vi "Measure Current.vi"(8 "error in":errorcluster, 11 "6700 in":refnum<class "6700.lvclass">) -> (0 "error out":errorcluster, 2 "Current":dbl, 3 "6700 out":refnum<class "6700.lvclass">)   [LabVIEW 2018, in "6700.lvlib" / "6700.lvclass"]
uses:
  6700.lvclass
  6700.lvclass/6700.ctl
  <instrlib>/Agilent N6700 Series/Agilent N6700 Series.lvlib
  builds/Power_Supply.lvlibp/Power Supply.lvclass
  C:/Users/Ron.Dexter.LUMINARTECH/Desktop/builds/Power_Supply.lvlibp/Power Supply.lvclass
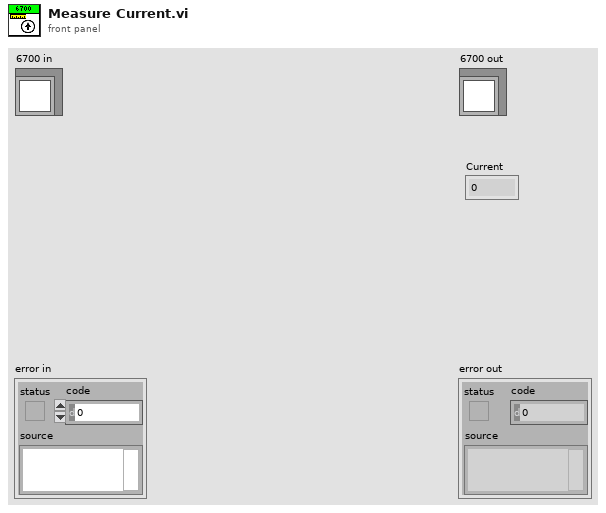
[diagram p1: front panel]
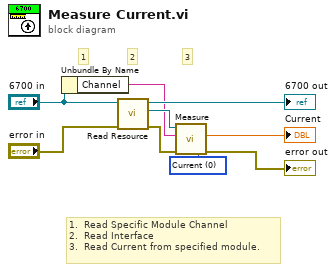
[diagram p0: block diagram]
diagram:
  w4 = 0 items=["Current", "Voltage", "Power"] ("Measurement Type (1: Voltage)")
  # "1.  Read Specific Module Channel \n2.  Read Interface\n3.  Read Current from specified module."
  # "3"
  # "2"
  # "1"
  n1 = Unbundle By Name("6700 in") -> ("Channel"=w1:string)
  n2 = call "Read Resource.vi"("error in"="error in", "Power Supply in"="6700 in") -> ("error out"=w5:errorcluster, "Resource"=w9:refnum<visa-resource-name>, "Power Supply out"=→"6700 out":refnum<class "6700.lvclass">)  [unwired: 7 in]
  n3 = call <instrlib>:"Measure.vi"("error in (no error)"=w5, "Measurement Type (1: Voltage)"=w4, "Channel Name (1)"=w1, "VISA resource name"=w9) -> ("error out"=→"error out":errorcluster, "Measurement"=→"Current":dbl)  [unwired: 5 in, 1 out]
